vi "nearCamSnapOnce.vi"() -> (0 "error out":errorcluster, 2 "Image Out":T1)   [LabVIEW 2018]
uses:
  <vilib>/vision/Image Controls.llb/IMAQ Image.ctl
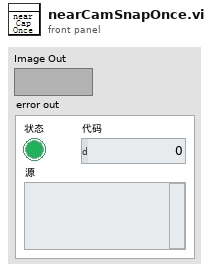
[diagram p1: front panel]
types:
  T1 = typedef "IMAQ Image.ctl" = refnum<image>
  T2 = cluster{"示波器":cluster{"Channel (0:Channel 1)":enum16{"Channel 1", "Channel 2", "Channel 3", "Channel 4"}, "电压范围":dbl, "触发电压":dbl, "时间范围":dbl, " 示波器VISA":refnum<visa-resource-name>, "时间范围 标签":u64, "电压范围 标签":u64, "触发电压 标签":u64, "输入阻抗/Ω":u64}, "光谱仪":cluster{"SpecDataReference":refnum<queue>, "grating center":dbl, "Exposure Time (s)":dbl, "是否进行详细设置":bool, " 开始通信检查":bool, "通信成功？":bool, "波长":dbl}, " 近场相机":cluster{"曝光时间/100us":dbl, "模拟增益":i32, "控制套接字":i32, "IP 地址":string, " 采集套接字":i32, "  版本号":i32, "ImageData":T1, "  增益最大":i32, "  增益最小":i32, " 曝光最大":i32, " 曝光最小":i32, " 帧速":i32, " 同步切换":i32, "  曝光缩放":i32}, " 偏振仪":cluster{"电压范围":u64, "触发电压":u64, "时间范围":u64, "波长范围":enum16{"可见光 400-700nm", "近红外 700-1100nm"}, "可见光偏振测量仪VISA":refnum<visa-resource-name>, "近红外偏振测量仪VISA":refnum<visa-resource-name>}, " 功率计":cluster{"通道":enum16{"Channel 1", "Channel 2"}, "工作波长":u32, "单位":u64, "时间范围":u64, "IP地址":string, "端口":u32}, "能量计":cluster{"通道":enum16{"Channel 1", "Channel 2"}, "工作波长":u32, "单位":u64, "时间范围":u64, "IP地址":string, "端口":u32, "能量计量程":enum16{"200uJ", "20uJ", "2uJ", "200nJ"}}, "电机":cluster{"Channel (0:Channel 1)":enum16{"Channel 1", "Channel 2", "Channel 3", "Channel 4"}, "电压范围":u64, "触发电压":u64, "时间范围":u64}, " 远场相机":cluster{"曝光时间":i32, "模拟增益":i32, "控制套接字":i32, "IP 地址":string, " 采集套接字":i32, "  版本号":i32, "ImageData":T1, "  增益最大":i32, "  增益最小":i32, " 曝光最大":i32, " 曝光最小":i32, " 帧速":i32, " 同步切换":i32, "  曝光缩放":i32, "ImageData B":T1}}
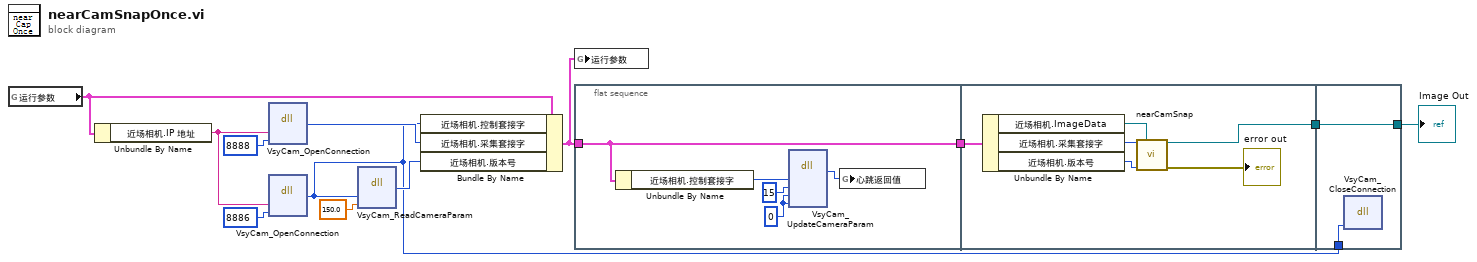
[diagram p0: block diagram]
diagram:
  n1 = global read "参数.vi" "运行参数"() -> (w4:T2)
  n2 = Unbundle By Name(w4) -> ("近场相机.IP 地址"=w8:string)
  n3 = dll-call lib="PTH2^abs E航天测量驱动相机驱动LabView2014Demo_V1.0.8\nLabView14Demo\nVsyCam.dll" fn="VsyCam_OpenConnection"("ip"=w8, "port"=8888) -> ("返回类型"=w6:i32)  [unwired: 5 in, 2 out]
  n4 = dll-call lib="PTH2^abs E航天测量驱动相机驱动LabView2014Demo_V1.0.8\nLabView14Demo\nVsyCam.dll" fn="VsyCam_OpenConnection"("ip"=w8, "port"=8886) -> ("返回类型"=w1:i32)  [unwired: 5 in, 2 out]
  n5 = dll-call lib="PTH2^abs E航天测量驱动相机驱动LabView2014Demo_V1.0.8\nLabView14Demo\nVsyCam.dll" fn="VsyCam_ReadCameraParam"("sockFd"=w1, "cmd"=150.0) -> ("返回类型"=w5:i32)  [unwired: 5 in, 2 out]
  n6 = Bundle By Name(cluster=w4, "近场相机.控制套接字"=w1, "近场相机.采集套接字"=w6, "近场相机.版本号"=w5) -> (w3:T2)
  n7 = global write "参数.vi" "运行参数"(w3) -> ()
  n8 = flat-sequence {
    tunnel: [w13] -> w11
    tunnel: w3 -> [w13]
    tunnel: w11 -> [w18]
    tunnel: [w20] -> w2
    tunnel: [w25] -> w12
    tunnel: w2 -> [w25]
    tunnel: w1 -> [w24]
    frame #0 {
      w14 = 0
      n9 = Unbundle By Name(w13) -> ("近场相机.控制套接字"=w17:i32)
      n10 = dll-call lib="PTH2^abs E航天测量驱动相机驱动LabView2014Demo_V1.0.8\nLabView14Demo\nVsyCam.dll" fn="VsyCam_UpdateCameraParam"("sockFd"=w17, "command"=15, "value"=w14, "ack"=w14) -> ("返回类型"=w16:i32)  [unwired: 7 in, 2 out]
      n11 = global write "globalMessage.vi" "心跳返回值"(w16) -> ()
    }
    frame #1 {
      n12 = Unbundle By Name(w18) -> ("近场相机.ImageData"=w23:T1, "近场相机.采集套接字"=w22:i32, "近场相机.版本号"=w21:i32)
      n13 = call "nearCamSnap.vi"("采集套接字"=w22, "ImageData"=w23, "版本号"=w21) -> ("Image Out"=w20:T1, "error out"=→"error out":errorcluster)  [unwired: 9 in, 2 out]
    }
    frame #2 {
      n14 = dll-call lib="PTH2^abs E航天测量驱动相机驱动LabView2014Demo_V1.0.8\nLabView14Demo\nVsyCam.dll" fn="VsyCam_CloseConnection"("sockFd"=w24) -> ()  [unwired: 5 in, 2 out]
    }
  }
  "Image Out" <- w12
